vi "Initialize-uv-visSD.vi"(2 "error in (no error)":errorcluster, 3 "directory (\"\")":string) -> (0 "error out":errorcluster, 1 "DLL error code":u32)   [LabVIEW 2015]
doc: "This function will initialize the AndorMCD[tm] System. As part of the initialization procedure the DLL will need access to three files. The first file is \"DETECTOR.INI\" which contains information relating to the detector head, number pixels, readout speeds etc. The second file has the extension \"COF\" and contains the run-time code for the microprocessor on the AndorMCD[tm] plug-in card. The third file has the extension \"RBF\" and contains data for the FPGA on the plug-in card. If \"directory\" is NULL or an empty string then the driver will search the current working directory for the files. If any of these files cannot be loaded then the system will NOT be able to acquire data.\n\n<B>Parameter:</B>\ndirectory - path to the directory containing the files\n\n<B>Error codes:</B>\nDRV_SUCCESS - System fully initialized.\nDRV_VXDNOTINSTALLED - VxD not loaded.\nDRV_INIERROR - Unable to load \"DETECTOR.INI\".\nDRV_COFERROR - Unable to load \"*.COF\".\nDRV_FLEXERROR - Unable to load \"*.RBF\".\nDRV_ERROR_ACK - Unable to communicate with card.\nDRV_ERROR_FILELOAD - Unable to load \"*.COF\" or \"*.RBF\" files.\nDRV_ERROR_PAGELOCK - Unable to acquire lock on requested memory.\n\n<B>NOTES:</B>\n<B>This function must be called first to ensure that the system is fully initialized.</B>"
uses:
  DLL/atmcd32d.dll
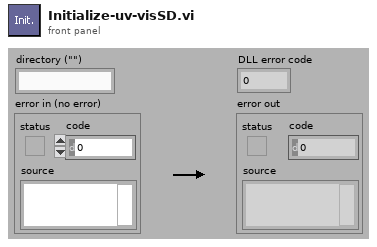
[diagram p1: front panel]
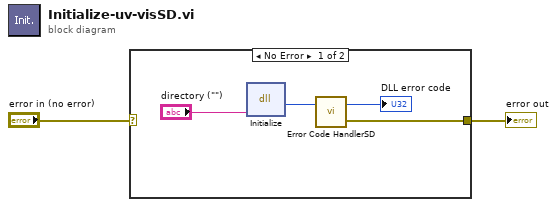
[diagram p0: block diagram]
diagram:
  n1 = case shown="No Error" "error in (no error)" {
    selector: "error in (no error)" -> [_ w7]
    tunnel: [w5 w7] -> w1
    frame No Error {
      n2 = dll-call lib="G:/SD/TRANCON-2015/DLL/Atmcd32d.dll" fn="Initialize"("directory"="directory (\"\")") -> (w6:u32)  [unwired: 4 in, 2 out]
      n3 = call "Error Code HandlerSD.vi"("DLL error code"=w6) -> ("error out"=w5:errorcluster, "dup DLL error code"=→"DLL error code":u32)  [unwired: 1 in]
    }
    frame Error {
    }
  }
  "error out" <- w1
